vi "iRobot Read Sensor Group 5.vi"(11 "stream in":u8[](array[numeric])) -> (1 "Sensor Group 5":T1, 3 "stream out":u8[](array[numeric]))   [LabVIEW 2010]
doc: "Read Sensor Group 5 from a UART data stream."
uses:
  Sensor Controls/iRobot Sensor Group 5.ctl
  Sensor Controls/iRobot OI Mode.ctl
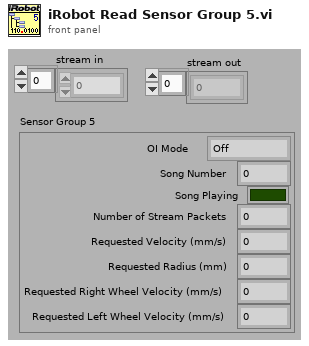
[diagram p1: front panel]
types:
  T1 = typedef "iRobot Sensor Group 5.ctl" = cluster{"OI Mode":T2, "Song Number":u8, "Song Playing":bool, "Number of Stream Packets":u8, "Requested Velocity (mm/s)":u8, "Requested Radius (mm)":u8, "Requested Right Wheel Velocity (mm/s)":u8, "Requested Left Wheel Velocity (mm/s)":u8}
  T2 = typedef "iRobot OI Mode.ctl" = enum16{"Off", "Passive", "Safe", "Full"}
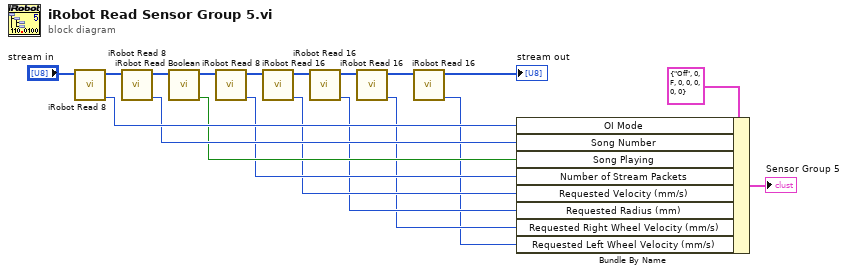
[diagram p0: block diagram]
diagram:
  n1 = call "iRobot Read 8.vi"("stream in"="stream in") -> ("value"=w16:u8, "stream out"=w15:u8[])  [unwired: 9 out]
  n2 = call "iRobot Read 8.vi"("stream in"=w15) -> ("value"=w14:u8, "stream out"=w13:u8[])  [unwired: 9 out]
  n3 = call "iRobot Read Boolean.vi"("stream in"=w13) -> ("Value"=w12:bool, "stream out"=w11:u8[])  [unwired: 9 out]
  n4 = call "iRobot Read 8.vi"("stream in"=w11) -> ("value"=w10:u8, "stream out"=w9:u8[])  [unwired: 9 out]
  n5 = call "iRobot Read 16.vi"("stream in"=w9) -> ("value"=w8:u16, "stream out"=w7:u8[])  [unwired: 9 out]
  n6 = call "iRobot Read 16.vi"("stream in"=w7) -> ("value"=w6:u16, "stream out"=w5:u8[])  [unwired: 9 out]
  n7 = call "iRobot Read 16.vi"("stream in"=w5) -> ("value"=w4:u16, "stream out"=w3:u8[])  [unwired: 9 out]
  n8 = call "iRobot Read 16.vi"("stream in"=w3) -> ("value"=w2:u16, "stream out"=→"stream out":u8[])  [unwired: 9 out]
  n9 = Bundle By Name(cluster=T1 {"OI Mode"=enum."Off", "Song Number"=0, "Song Playing"=FALSE, "Number of Stream Packets"=0, "Requested Velocity (mm/s)"=0, "Requested Radius (mm)"=0, "Requested Right Wheel Velocity (mm/s)"=0, "Requested Left Wheel Velocity (mm/s)"=0} ("Sensor Group 5"), "OI Mode"=w16, "Song Number"=w14, "Song Playing"=w12, "Number of Stream Packets"=w10, "Requested Velocity (mm/s)"=w8, "Requested Radius (mm)"=w6, "Requested Right Wheel Velocity (mm/s)"=w4, "Requested Left Wheel Velocity (mm/s)"=w2) -> (→"Sensor Group 5":T1)
